vi "LoadGCSFromSingleLLB.vi"(11 "LLB containing GCS VIs":path) -> (3 "PI GCS Function\nReferences":T1)   [LabVIEW 2011]
uses:
  GCS_Interface.ctl
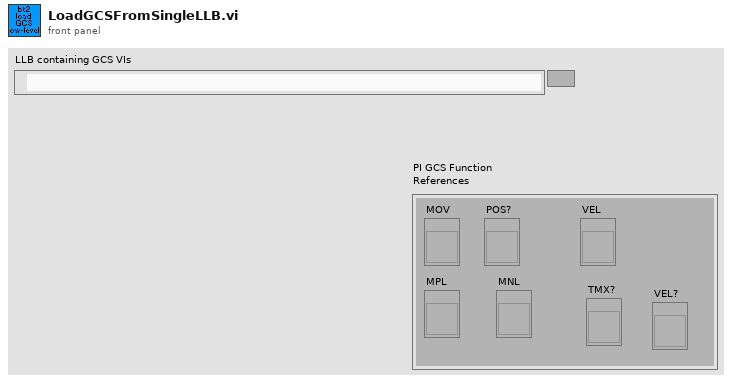
[diagram p1: front panel]
types:
  T1 = typedef "GCS_Interface.ctl" = cluster{"MOV":refnum<vi>, "VEL":refnum<vi>, "VEL?":refnum<vi>, "POS?":refnum<vi>, "TMX?":refnum<vi>, "MPL":refnum<vi>, "MNL":refnum<vi>}
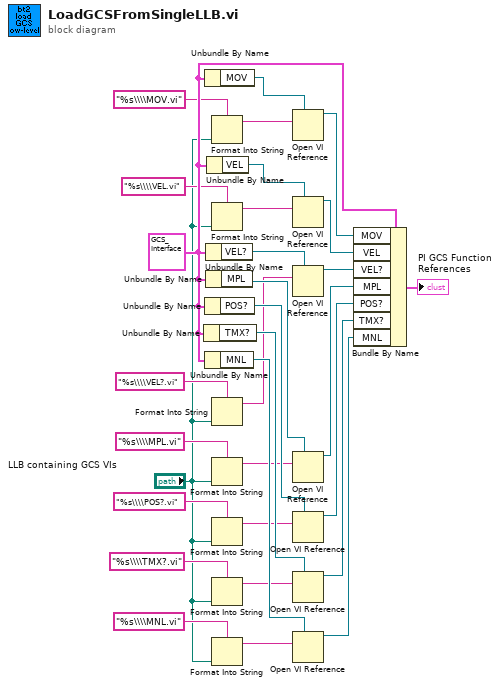
[diagram p0: block diagram]
diagram:
  w17 = T1 {"MOV"=refnum, "VEL"=refnum, "VEL?"=refnum, "POS?"=refnum, "TMX?"=refnum, "MPL"=refnum, "MNL"=refnum} ("PI GCS Function\nReferences")
  n1 = Unbundle By Name(w17) -> ("TMX?"=w29:refnum<vi>)
  n2 = Unbundle By Name(w17) -> ("MOV"=w21:refnum<vi>)
  n3 = Unbundle By Name(w17) -> ("POS?"=w16:refnum<vi>)
  n4 = Unbundle By Name(w17) -> ("MNL"=w23:refnum<vi>)
  n5 = Unbundle By Name(w17) -> ("VEL?"=w19:refnum<vi>)
  n6 = Unbundle By Name(w17) -> ("MPL"=w18:refnum<vi>)
  n7 = Unbundle By Name(w17) -> ("VEL"=w20:refnum<vi>)
  n8 = Format Into String(format string="%s\\\\MOV.vi", "LLB containing GCS VIs") -> (resulting string=w14:string)  [unwired: 2 in, 1 out]
  n9 = Format Into String(format string="%s\\\\VEL.vi" ("name or relative path"), "LLB containing GCS VIs") -> (resulting string=w11:string)  [unwired: 2 in, 1 out]
  n10 = Format Into String(format string="%s\\\\VEL?.vi" ("name or relative path"), "LLB containing GCS VIs") -> (resulting string=w10:string)  [unwired: 2 in, 1 out]
  n11 = Format Into String(format string="%s\\\\MPL.vi" ("name or relative path"), "LLB containing GCS VIs") -> (resulting string=w9:string)  [unwired: 2 in, 1 out]
  n12 = Format Into String(format string="%s\\\\POS?.vi" ("name or relative path"), "LLB containing GCS VIs") -> (resulting string=w6:string)  [unwired: 2 in, 1 out]
  n13 = Format Into String(format string="%s\\\\TMX?.vi" ("name or relative path"), "LLB containing GCS VIs") -> (resulting string=w4:string)  [unwired: 2 in, 1 out]
  n14 = Format Into String(format string="%s\\\\MNL.vi" ("name or relative path"), "LLB containing GCS VIs") -> (resulting string=w1:string)  [unwired: 2 in, 1 out]
  n15 = Open VI Reference(type specifier VI Refnum (for type only)=w21, vi path=w14) -> (vi reference=w30:refnum<vi>)  [unwired: 4 in, 1 out]
  n16 = Open VI Reference(type specifier VI Refnum (for type only)=w20, vi path=w11) -> (vi reference=w27:refnum<vi>)  [unwired: 4 in, 1 out]
  n17 = Open VI Reference(type specifier VI Refnum (for type only)=w19, vi path=w10) -> (vi reference=w26:refnum<vi>)  [unwired: 4 in, 1 out]
  n18 = Open VI Reference(type specifier VI Refnum (for type only)=w18, vi path=w9) -> (vi reference=w24:refnum<vi>)  [unwired: 4 in, 1 out]
  n19 = Open VI Reference(type specifier VI Refnum (for type only)=w16, vi path=w6) -> (vi reference=w28:refnum<vi>)  [unwired: 4 in, 1 out]
  n20 = Open VI Reference(type specifier VI Refnum (for type only)=w29, vi path=w4) -> (vi reference=w25:refnum<vi>)  [unwired: 4 in, 1 out]
  n21 = Open VI Reference(type specifier VI Refnum (for type only)=w23, vi path=w1) -> (vi reference=w22:refnum<vi>)  [unwired: 4 in, 1 out]
  n22 = Bundle By Name(cluster=w17, "MOV"=w30, "VEL"=w27, "VEL?"=w26, "MPL"=w24, "POS?"=w28, "TMX?"=w25, "MNL"=w22) -> (→"PI GCS Function\nReferences":T1)
